vi "ATF-Storage-Index getter  Digital.vi"(9 "output cluster":T1, 10 "DI Y  data":bool[](array[boolean]), 11 "DI Channels Name":string[](array[string])) -> (3 "Digital data":bool)   [LabVIEW 2022 SP3]
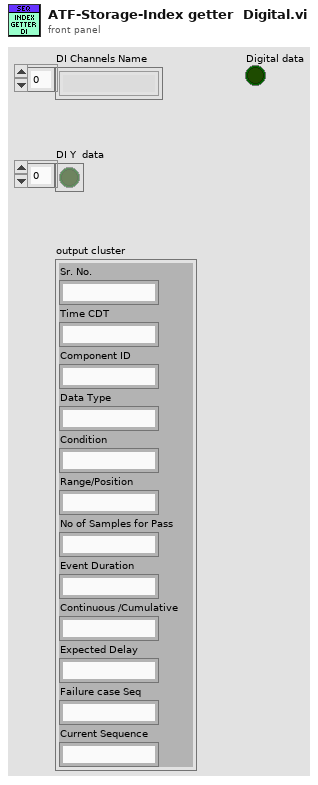
[diagram p1: front panel]
types:
  T1 = cluster{"Sr. No.":string, "Time CDT":string, "Component ID":string, "Data Type":string, "Condition":string, "Range/Position":string, "No of Samples for Pass":string, "Event Duration":string, "Continuous /Cumulative":string, "Expected Delay":string, "Failure case Seq":string, "Current Sequence":string}
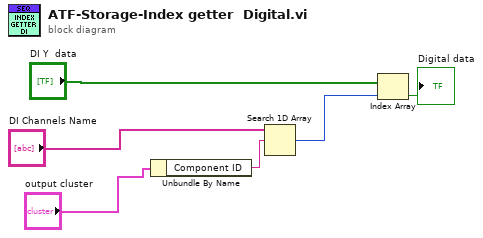
[diagram p0: block diagram]
diagram:
  n1 = Unbundle By Name("output cluster") -> ("Component ID"=w2:string)
  n2 = Search 1D Array(1D array="DI Channels Name", element=w2) -> (index of element=w6:i32)  [unwired: 1 in]
  n3 = Index Array(array="DI Y  data", index=w6) -> (element=→"Digital data":bool)
